vi "Invert Channel Direction.vi"(11 "Channels to Create":T1[](array[typedef]) {"Custom Config Data" format="%x"}) -> (3 "Inverted Channels to Create":T1[](array[typedef]) {"Custom Config Data" format="%x"})   [LabVIEW 2021, in "Template_Test_Helpers.lvlib"]
uses:
  Template_Test_Helpers.lvlib
  <vilib>/CIF Foundation/CIF Core/Channels/ChannelRegistrar/typedef/Channel Definition.ctl
  <vilib>/CIF Foundation/CIF Channels Core/ChannelCommon/typedef/Direction.ctl
  <vilib>/CIF Foundation/CIF Core/Channels/ChannelRegistrar/typedef/Registered Channel Types.ctl
  <vilib>/CIF Foundation/CIF Channels Core/ChannelCommon/ChannelCommon.lvlib
  <vilib>/CIF Foundation/CIF Core/Channels/ChannelRegistrar/ChannelRegistrar.lvlib
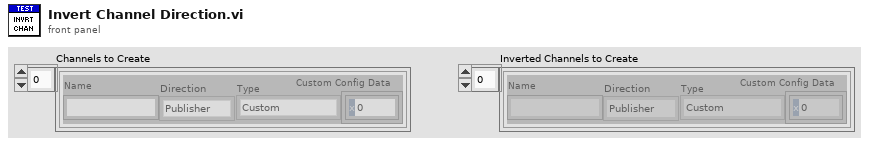
[diagram p1: front panel]
types:
  T1 = typedef "ChannelRegistrar.lvlib/Channel Definition.ctl" = cluster{"Name":string, "Direction":T2, "Type":T3, "Custom Config Data":u8[]}
  T2 = typedef "ChannelCommon.lvlib/Direction.ctl" = enum8{"Publisher", "Subscriber"}
  T3 = typedef "ChannelRegistrar.lvlib/Registered Channel Types.ctl" = enum8{"Custom", "Double_Tag", "I64_Tag", "U64_Tag", "U8_FIFO", "CAN_FIFO", "L2Enet_FIFO", "DAQ_FIFO", "Universal_FIFO", "String_Tag"}
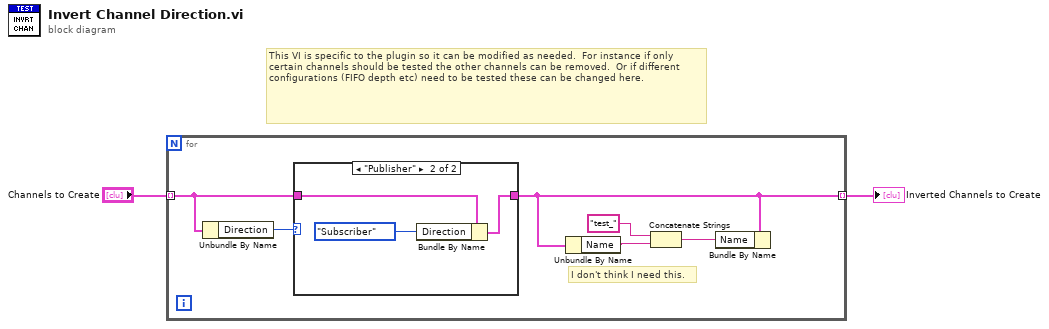
[diagram p0: block diagram]
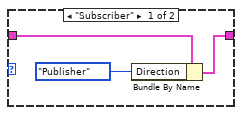
[diagram p2: hidden frame]
diagram:
  # "This VI is specific to the plugin so it can be modified as needed.  For instance if only certain channels should be tested the other channels can be removed.  Or if different configurations (FIFO depth etc) need to be tested these can be changed here."
  n1 = for {
    tunnel: "Channels to Create" -> [w7] mode=indexing
    tunnel: [w3] -> w2 mode=indexing
    # "I don't think I need this."
    n2 = Unbundle By Name(w7) -> ("Direction"=w8:T2)
    n3 = case shown="\"Publisher\"" w8 {
      tunnel: w7 -> [w11 w14]
      tunnel: [w9 w12] -> w3
      frame "Subscriber" {
        n4 = Bundle By Name(cluster=w11, "Direction"=Direction."Publisher") -> (w9:T1)
      }
      frame "Publisher" {
        n5 = Bundle By Name(cluster=w14, "Direction"=Direction."Subscriber") -> (w12:T1)
      }
    }
    n6 = Unbundle By Name(w3) -> ("Name"=w6:string)
    n7 = Concatenate Strings("test_" ("string"), w6) -> (w4:string)
    n8 = Bundle By Name(cluster=w3, "Name"=w4) -> ()  [unwired: 1 out]
  }
  "Inverted Channels to Create" <- w2
